vi "Auto Transmission read constants.vi"(8 "error in (no error)":errorcluster) -> (0 "error out":errorcluster, 3 "All Shifter Constants":T1)   [LabVIEW 2013]
uses:
  All Shifter Constants.ctl
  Shift Constants.ctl
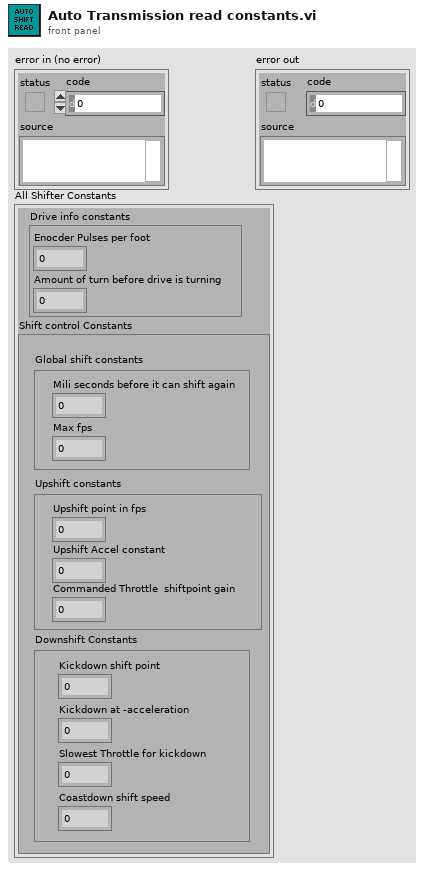
[diagram p1: front panel]
types:
  T1 = typedef "All Shifter Constants.ctl" = cluster{"Drive info constants":cluster{"Enocder Pulses per foot":dbl, "Amount of turn before drive is turning":dbl}, "Shift control Constants":T2}
  T2 = typedef "Shift Constants.ctl" = cluster{"Global shift constants":cluster{"Mili seconds before it can shift again":u32, "Max fps":dbl}, "Upshift constants":cluster{"Upshift point in fps":dbl, "Upshift Accel constant":dbl, "Commanded Throttle  shiftpoint gain":dbl}, "Downshift Constants":cluster{"Kickdown shift point":dbl, "Kickdown at -acceleration":dbl, "Slowest Throttle for kickdown":dbl, "Coastdown shift speed":dbl}}
  T3 = cluster{"Enocder Pulses per foot":dbl, "Amount of turn before drive is turning":dbl}
  T4 = cluster{"Mili seconds before it can shift again":u32, "Max fps":dbl}
  T5 = cluster{"Upshift point in fps":dbl, "Upshift Accel constant":dbl, "Commanded Throttle  shiftpoint gain":dbl}
  T6 = cluster{"Kickdown shift point":dbl, "Kickdown at -acceleration":dbl, "Slowest Throttle for kickdown":dbl, "Coastdown shift speed":dbl}
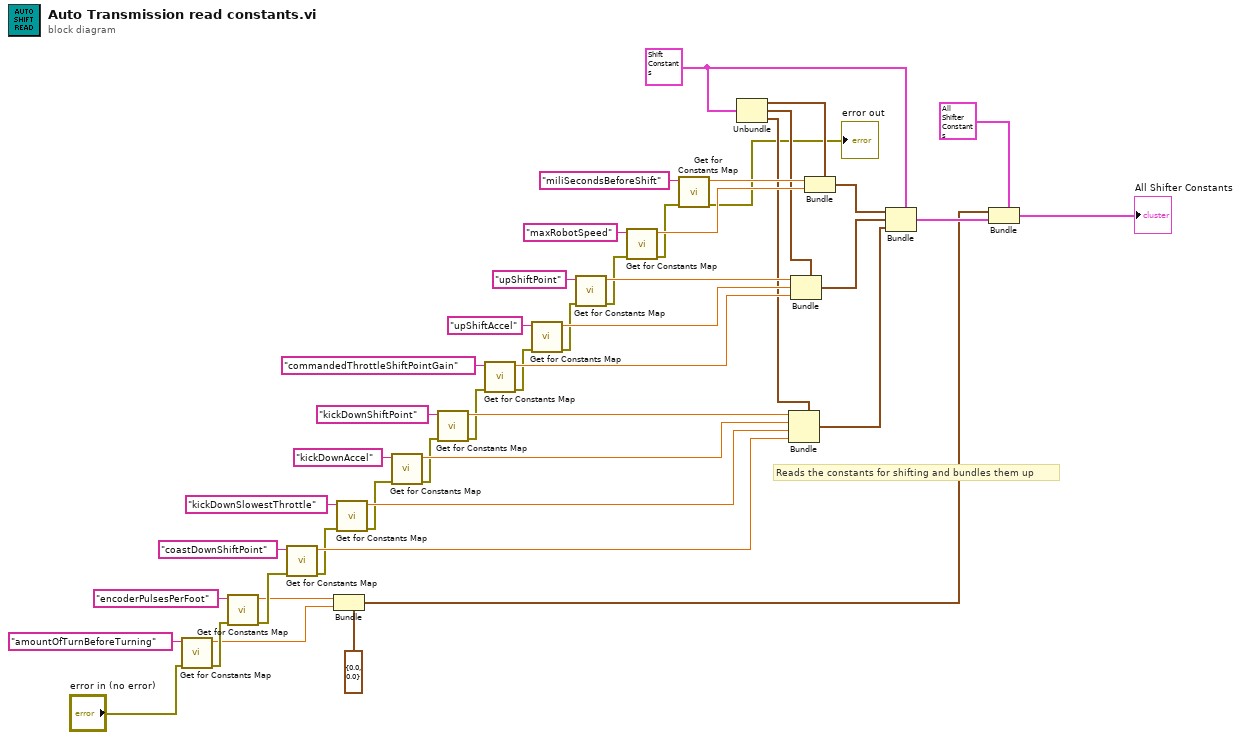
[diagram p0: block diagram]
diagram:
  w46 = T2 {"Global shift constants"={"Mili seconds before it can shift again"=0, "Max fps"=0.0}, "Upshift constants"={"Upshift point in fps"=0.0, "Upshift Accel constant"=0.0, "Commanded Throttle  shiftpoint gain"=0.0}, "Downshift Constants"={"Kickdown shift point"=0.0, "Kickdown at -acceleration"=0.0, "Slowest Throttle for kickdown"=0.0, "Coastdown shift speed"=0.0}} ("Shift Constants 2")
  # "Reads the constants for shifting and bundles them up"
  n1 = call "Get for Constants Map.vi"("error in (no error)"="error in (no error)", "Constant Name"="amountOfTurnBeforeTurning") -> ("error out"=w7:errorcluster, "Value"=w1:dbl)  [unwired: 7 in, 1 out]
  n2 = call "Get for Constants Map.vi"("error in (no error)"=w7, "Constant Name"="encoderPulsesPerFoot") -> ("error out"=w8:errorcluster, "Value"=w2:dbl)  [unwired: 7 in, 1 out]
  n3 = call "Get for Constants Map.vi"("error in (no error)"=w8, "Constant Name"="coastDownShiftPoint") -> ("error out"=w14:errorcluster, "Value"=w22:dbl)  [unwired: 7 in, 1 out]
  n4 = Bundle(cluster=T3 {"Enocder Pulses per foot"=0.0, "Amount of turn before drive is turning"=0.0} ("Drive info constants"), "Enocder Pulses per foot"=w2, "Amount of turn before drive is turning"=w1) -> (w3:T3)
  n5 = call "Get for Constants Map.vi"("error in (no error)"=w14, "Constant Name"="kickDownSlowestThrottle") -> ("error out"=w15:errorcluster, "Value"=w23:dbl)  [unwired: 7 in, 1 out]
  n6 = call "Get for Constants Map.vi"("error in (no error)"=w15, "Constant Name"="kickDownAccel") -> ("error out"=w16:errorcluster, "Value"=w24:dbl)  [unwired: 7 in, 1 out]
  n7 = call "Get for Constants Map.vi"("error in (no error)"=w16, "Constant Name"="kickDownShiftPoint") -> ("error out"=w17:errorcluster, "Value"=w26:dbl)  [unwired: 7 in, 1 out]
  n8 = call "Get for Constants Map.vi"("error in (no error)"=w17, "Constant Name"="commandedThrottleShiftPointGain") -> ("error out"=w18:errorcluster, "Value"=w33:dbl)  [unwired: 7 in, 1 out]
  n9 = call "Get for Constants Map.vi"("error in (no error)"=w18, "Constant Name"="upShiftAccel") -> ("error out"=w19:errorcluster, "Value"=w35:dbl)  [unwired: 7 in, 1 out]
  n10 = call "Get for Constants Map.vi"("error in (no error)"=w19, "Constant Name"="upShiftPoint") -> ("error out"=w20:errorcluster, "Value"=w37:dbl)  [unwired: 7 in, 1 out]
  n11 = call "Get for Constants Map.vi"("error in (no error)"=w20, "Constant Name"="maxRobotSpeed") -> ("error out"=w21:errorcluster, "Value"=w41:dbl)  [unwired: 7 in, 1 out]
  n12 = call "Get for Constants Map.vi"("error in (no error)"=w21, "Constant Name"="miliSecondsBeforeShift") -> ("error out"=→"error out":errorcluster, "Value"=w44:dbl)  [unwired: 7 in, 1 out]
  n13 = Unbundle(w46) -> ("Global shift constants"=w45:T4, "Upshift constants"=w39:T5, "Downshift Constants"=w31:T6)
  n14 = Bundle(cluster=w31, "Kickdown shift point"=w26, "Kickdown at -acceleration"=w24, "Slowest Throttle for kickdown"=w23, "Coastdown shift speed"=w22) -> (w25:T6)
  n15 = Bundle(cluster=w39, "Upshift point in fps"=w37, "Upshift Accel constant"=w35, "Commanded Throttle  shiftpoint gain"=w33) -> (w32:T5)
  n16 = Bundle(cluster=w45, "Mili seconds before it can shift again"=w44, "Max fps"=w41) -> (w40:T4)
  n17 = Bundle(cluster=w46, "Global shift constants"=w40, "Upshift constants"=w32, "Downshift Constants"=w25) -> (w11:T2)
  n18 = Bundle(cluster=T1 {"Drive info constants"={"Enocder Pulses per foot"=0.0, "Amount of turn before drive is turning"=0.0}, "Shift control Constants"={"Global shift constants"={"Mili seconds before it can shift again"=0, "Max fps"=0.0}, "Upshift constants"={"Upshift point in fps"=0.0, "Upshift Accel constant"=0.0, "Commanded Throttle  shiftpoint gain"=0.0}, "Downshift Constants"={"Kickdown shift point"=0.0, "Kickdown at -acceleration"=0.0, "Slowest Throttle for kickdown"=0.0, "Coastdown shift speed"=0.0}}} ("All Shifter Constants 2"), "Drive info constants"=w3, "Shift control Constants"=w11) -> (→"All Shifter Constants":T1)
